vi "setChillerStatus.vi"(8 "error in (no error)":errorcluster, 10 "ChillerStatus in":T2, 11 "CoolerControler in":refnum<class "CoolerControler.lvclass">) -> (0 "error out":errorcluster, 2 "ChillerStatus out":T2, 3 "CoolerControler out":refnum<class "CoolerControler.lvclass">)   [LabVIEW 2016, in "CoolerControler.lvclass"]
uses:
  CoolerControler.lvclass
  typedefs/ChillerStatus.ctl
  typedefs/CoolerId.ctl
  SerialCommand/CoolerSerialCommand.lvclass
  typedefs/dataUnit.ctl
  typedefs/CoolerCommands.ctl
panel:
  in  "id":T1=1
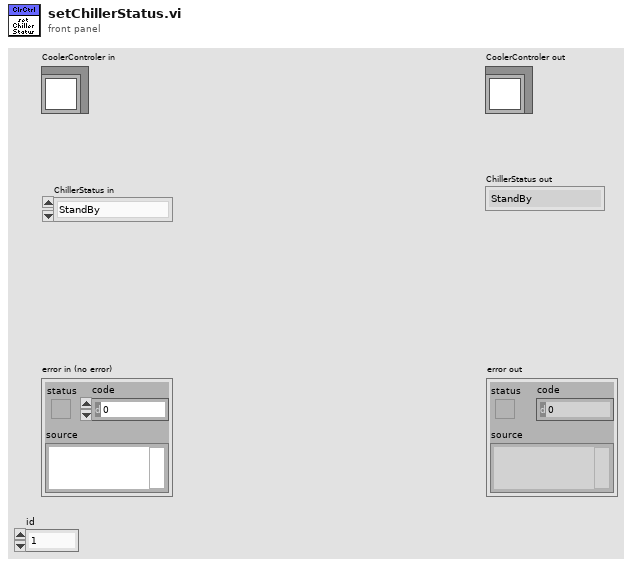
[diagram p1: front panel]
types:
  T1 = typedef "CoolerId.ctl" = u16
  T2 = typedef "ChillerStatus.ctl" = enum16{"StandBy", "Run"}
  T3 = typedef "CoolerCommands.ctl" = enum16{"None", "SetExternSensorStatus", "SetChillerStatus", "SetControlSensor", "SetControlTemperature", "SetHighSupplyTempWarning", "SetLowSupplyTemperatureWarning", "SetHighAmbientTemperatureWarning", "SetLowAmbienTemperatureWarning", "SetLowProcessFlowWarning", "SetHighSupplyTemperatureAlarm", "SetLowSupplyTemperatureAlarm", "SetHighAmbientTemperatureAlarm", "SetLowAmbientTemperatureAlarm", "SetLowProcessFlowAlarm"}
  T4 = typedef "dataUnit.ctl" = enum16{"temperature", "flow", "current", "PID", "fanSpeed", "time", "PWM", "TEDriveLevel", "Number"}
  T5 = typedef "response.ctl" = cluster{"deviceId":string, "commandNumber":string, "errorActive":bool, "commandName":string, "responseData":string, "checkSum":string}
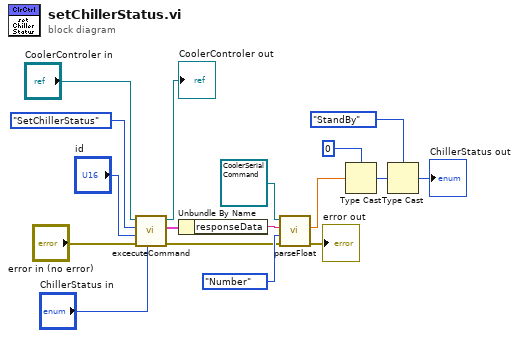
[diagram p0: block diagram]
diagram:
  n1 = call "excecuteCommand.vi"("inputValue"="ChillerStatus in", "error in (no error)"="error in (no error)", "id"="id", "CoolerCommand"=CoolerCommands."SetChillerStatus", "CoolerControler in"="CoolerControler in") -> ("error out"=w14:errorcluster, "response out"=w15:T5, "CoolerControler out"=→"CoolerControler out":refnum<class "CoolerControler.lvclass">)  [unwired: 4 in]
  n2 = Unbundle By Name(w15) -> ("responseData"=w17:string)
  n3 = call "parseFloat.vi"("error in (no error)"=w14, "unit"=dataUnit."Number", "commandData"=w17, "CoolerSerialCommand in"=refnum<class "CoolerSerialCommand.lvclass"> refnum) -> ("error out"=→"error out":errorcluster, "value"=w6:sgl)  [unwired: 4 in, 2 out]
  n4 = Type Cast(type=u16 0, x=w6) -> (*(type *) &x=w5:u16)
  n5 = Type Cast(type=ChillerStatus."StandBy" ("ChillerStatus out"), x=w5) -> (*(type *) &x=→"ChillerStatus out":T2)
